vi "Keithley24xx_MeasVil.vi"(0 "inVISA In":refnum<visa-resource-name>, 1 "Voh, V":dbl, 5 "outVISA In":refnum<visa-resource-name>, 7 "MeasF Out":string, 9 "Step, V":dbl, 11 "inErrI n":errorcluster, 12 "outErr In":errorcluster, 13 "Begin Level, V":dbl, 14 "Vil, V":dbl) -> (4 "outVISA Out":refnum<visa-resource-name>, 6 "inVISA Out":refnum<visa-resource-name>, 8 "Vil meas, В":dbl format="%#.3g", 10 "inErr Out":errorcluster, 15 "outErr Out":errorcluster)   [LabVIEW 2014]
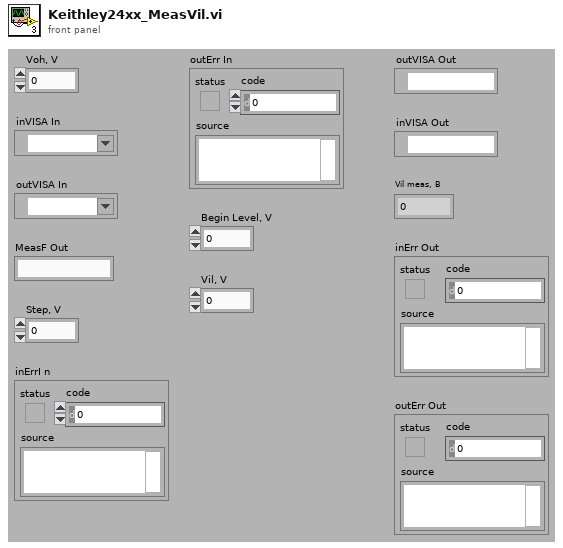
[diagram p1: front panel]
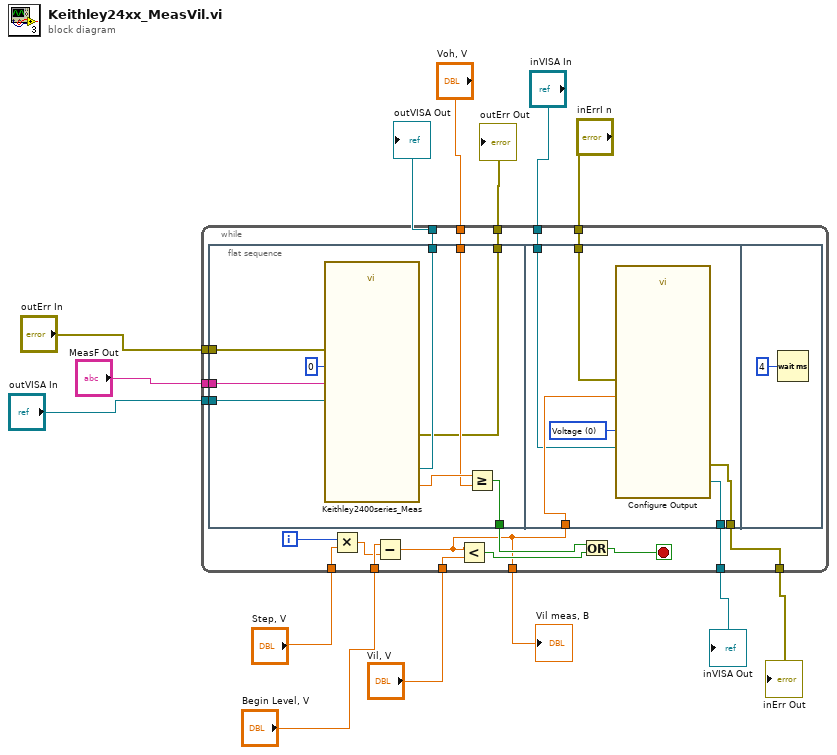
[diagram p0: block diagram]
diagram:
  n1 = while {
    tunnel: [w29] -> w8
    tunnel: "outErr In" -> [w28]
    tunnel: "MeasF Out" -> [w27]
    tunnel: "outVISA In" -> [w26]
    tunnel: "inErrI n" -> [w25]
    tunnel: "inVISA In" -> [w24]
    tunnel: "Step, V" -> [w23]
    tunnel: "Vil, V" -> [w22]
    tunnel: "Voh, V" -> [w21]
    tunnel: [w20] -> w6
    tunnel: [w19] -> w5
    tunnel: [w18] -> w4
    tunnel: [w17] -> w3
    tunnel: "Begin Level, V" -> [w16]
    i -> [w33]
    stop <- w30 stop-if-true
    n2 = flat-sequence {
      tunnel: [w41] -> w32
      tunnel: w28 -> [w39]
      tunnel: w27 -> [w38]
      tunnel: w26 -> [w37]
      tunnel: w21 -> [w36]
      tunnel: [w35] -> w20
      tunnel: [w34] -> w17
      tunnel: w29 -> [w47]
      tunnel: w25 -> [w46]
      tunnel: w24 -> [w45]
      tunnel: [w44] -> w19
      tunnel: [w43] -> w18
      frame #0 {
        n3 = call "Keithley2400series_Meas.vi"("MEAS:<f>"=w38, "error in (no error)"=w39, "MEAS mode, 0 Volt"=u16 0, "VISA resource name in"=w37) -> ("error out"=w34:errorcluster, "Замер"=w42:dbl, "VISA out"=w35:refnum<visa-resource-name>)  [unwired: 1 in, 1 out]
        n4 = Greater Or Equal?(x=w42, y=w36) -> (x >= y?=w41:bool)
      }
      frame #1 {
        w48 = u16 0 items=["Voltage", "Current"] ("Source Mode  (0: Voltage)")
        n5 = call "Configure Output.vi"("Source Mode  (0: Voltage)"=w48, "error in (no error)"=w46, "Output Level (0)"=w47, "VISA resource name"=w45) -> ("error out"=w43:errorcluster, "VISA resource name out"=w44:refnum<visa-resource-name>)  [unwired: 6 in]
      }
      frame #2 {
        n6 = Wait (ms)(milliseconds to wait=u32 4) -> ()  [unwired: 1 out]
      }
    }
    n7 = Multiply(x=w33, y=w23) -> (x*y=w15:dbl)
    n8 = Subtract(x=w16, y=w15) -> (x-y=w29:dbl)
    n9 = Less?(x=w29, y=w22) -> (x < y?=w31:bool)
    n10 = Or(x=w32, y=w31) -> (x .or. y?=w30:bool)
  }
  "Vil meas, В" <- w8
  "outVISA Out" <- w6
  "inVISA Out" <- w5
  "inErr Out" <- w4
  "outErr Out" <- w3
